vi "Test joystick.vi"() -> ()   [LabVIEW 2017]
uses:
  <vilib>/Utility/inputDevices.llb/closeJoystick.vi
panel:
  out "error out":errorcluster
  out "cluster":T1
  in  "stop":bool
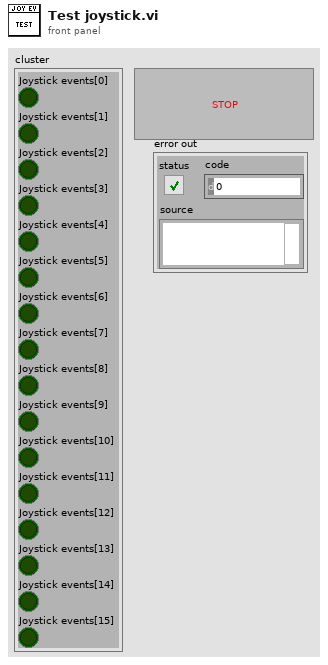
[diagram p1: front panel]
types:
  T1 = cluster{"Joystick events[0]":bool, "Joystick events[1]":bool, "Joystick events[2]":bool, "Joystick events[3]":bool, "Joystick events[4]":bool, "Joystick events[5]":bool, "Joystick events[6]":bool, "Joystick events[7]":bool, "Joystick events[8]":bool, "Joystick events[9]":bool, "Joystick events[10]":bool, "Joystick events[11]":bool, "Joystick events[12]":bool, "Joystick events[13]":bool, "Joystick events[14]":bool, "Joystick events[15]":bool}
  T2 = enum32{"Invalid", "Standard", "Closed", "Hidden", "Minimized", "Maximized"}
  T3 = typedef "Joystick event.ctl" = refnum<user-event>
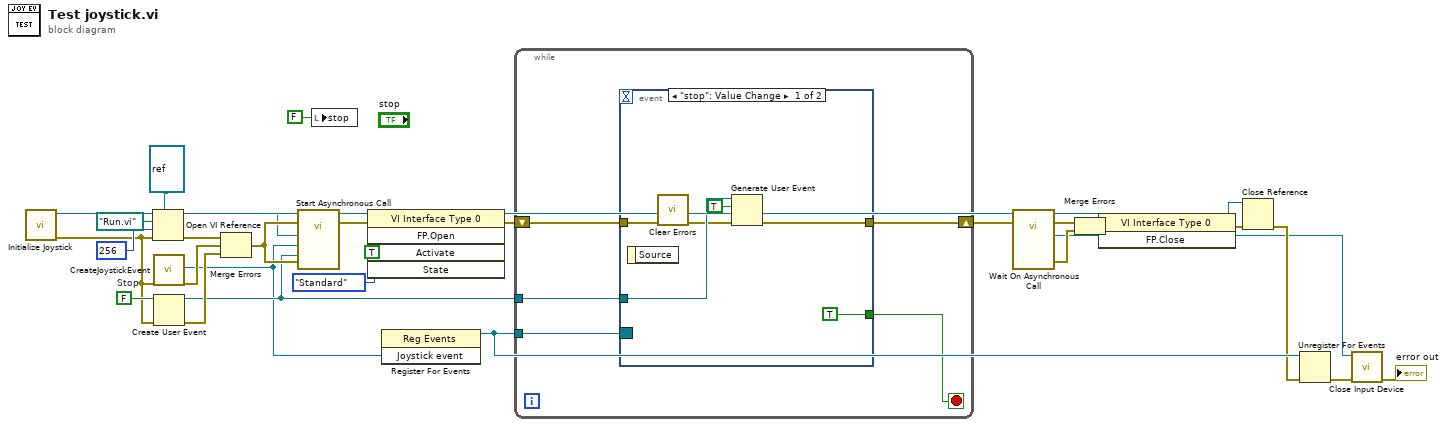
[diagram p0: block diagram]
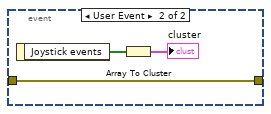
[diagram p2: hidden frame]
diagram:
  w28 = FALSE  # Stop
  n1 = call <vilib>:"Initialize Joystick.vi"() -> ("error out"=w4:errorcluster, "device ID"=w5:refnum<k1>)  [unwired: 10 in]
  n2 = Open VI Reference(type specifier VI Refnum (for type only)=refnum<vi> refnum, vi path=path "Run.vi", options=256, error in (no error)=w4) -> (vi reference=w29:refnum<vi>, error out=w13:errorcluster)  [unwired: 2 in]
  n3 = call "CreateJoystickEvent.vi"("error in"=w4) -> ("Joystick event"=w10:T3, "error out"=w15:errorcluster)  [unwired: 17 in]
  n4 = Create User Event(user event datatype=w28, error in=w4) -> (user event=w11:refnum<user-event>, error out=w14:errorcluster)
  n5 = Merge Errors(w13, w15, w14) -> (w12:errorcluster)
  n6 = call-by-ref "Start Asynchronous Call"(reference=w29, error in=w12, "Joystick ID"=w5, "Joystick event"=w10, "Stop event"=w11, "error in"=w12) -> (reference out=w26:refnum<vi>, error out=w25:errorcluster)  [unwired: 14 in, 2 out]
  n7 = local write "stop"(FALSE ("stop")) -> ()
  n8 = invoke class="VI Interface Type 0" method="FP.Open"(reference=w26, error in=w25, "Activate"=TRUE ("Activate?"), "State"=T2."Standard") -> (reference out=w7:refnum<vi>, error out=w17:errorcluster)  [unwired: 1 in, 3 out]
  n9 = register-events(w10) -> (reference out=w9:refnum<event-registration>)  [unwired: 2 in, 1 out]
  n10 = while {
    shift-right: [w36] -> w16
    shift-left: w17 -> [w37]
    tunnel: w11 -> [w35]
    tunnel: w9 -> [w33]
    stop <- w34 stop-if-true
    n11 = event shown="[0] \"stop\": Value Change" {
      selector: w33 -> [_ _]
      dyn-events: _ -> [_ _]
      timeout: _ -> [_ _]
      tunnel: w37 -> [w39 w46]
      tunnel: [w43 w46] -> w36
      tunnel: w35 -> [w42 _]
      tunnel: [TRUE _] -> w34
      event "stop": Value Change {
        n12 = event-data() -> ()  [unwired: 1 in, 1 out]
        n13 = call <vilib>:"Clear Errors.vi"("error in (no error)"=w39) -> ("error out"=w38:errorcluster)  [unwired: 5 in, 1 out]
        n14 = Generate User Event(user event=w42, event data cluster=TRUE ("event data"), error in=w38) -> (error out=w43:errorcluster)  [unwired: 1 in, 1 out]
      }
      event User Event {
        n15 = event-data() -> ("Joystick events"=w45:bool[])  [unwired: 1 in]
        n16 = Array To Cluster(array=w45) -> (cluster=→"cluster":T1)
      }
    }
  }
  n17 = call-by-ref "Wait On Asynchronous Call"(reference=w7, error in=w16) -> (reference out=w21:refnum<vi>, error out=w22:errorcluster, "Joystick ID out"=w1:refnum<k1>, 19:"error out"=w23:errorcluster)  [unwired: 18 in]
  n18 = Merge Errors(w22, w23) -> (w20:errorcluster)
  n19 = invoke class="VI Interface Type 0" method="FP.Close"(reference=w21, error in=w20) -> (reference out=w19:refnum<vi>, error out=w18:errorcluster)  [unwired: 1 in, 1 out]
  n20 = Close Reference(reference=w19, error in (no error)=w18) -> (error out=w8:errorcluster)
  n21 = Unregister For Events(event registration refnum=w9, error in=w8) -> (error out=w3:errorcluster)
  n22 = call-poly <vilib>:"Close Input Device.vi"("error in (no error)"=w3, "device ID"=w1) -> ("error out"=→"error out":errorcluster)  [unwired: 8 in]
